vi "Speed of VIight FPGA_v2.vi"() -> ()   [LabVIEW 2026]
uses:
  <vilib>/eio/EIONode/EIONode.xnode
  <vilib>/rvi/eio/common/nirviEmuTemplateMethod_errors.vi
  <instrlib>/_niInstr/Basic Elements/v1/FPGA/niInstr Basic Elements v1 FPGA.lvlib
  <instrlib>/_niInstr/Basic Elements/v1/FPGA/Private/Count Up U16.vi
panel:
  out "Any Invalid press":bool
  out "Any Press":bool
  out "Any Valid press":bool
  out "Idle Loop":i32
  in  "Period":u16=100
  in  "Idle Pattern":u16[](array[numeric])=[0, 0, 0, 0, 0, 0, 0, 0, 0, 0, 0, 0, 0, 0, 0, 0, 0, 0, 0, 0, 0, 0, 0, 0, 0, 0, 0, 0, 0, 0, 0, 0, 0, 0, 0, 0, 0, 0, 0, 0, 0, 0, 0, 0, 0]
  out "Main Loop Complete":bool
  out "Player 2 Output 5":bool[](array[boolean])
  out "Player 1 Output 5":bool[](array[boolean])
  out "Initial 6 Random Numbers":u8[](array[numeric])
  out "Player 2 Bonus":u8
  out "Player 1 Bonus":u8
  in  "Max Bonus":u8=5
  in  "Bonus Threshold":u64=3000
  out "Intial Random Arrays":u8[](array[numeric])
  out "Player2 Input":bool[](array[boolean])
  out "Player1 Input":bool[](array[boolean])
  out "Player 2 Output 4":bool[](array[boolean])
  out "Player 2 Output 3":bool[](array[boolean])
  out "Player 2 Output 2":bool[](array[boolean])
  out "Player 2 Output 1":bool[](array[boolean])
  out "Player 1 Output 4":bool[](array[boolean])
  out "Player 1 Output 3":bool[](array[boolean])
  out "Player 1 Output 2":bool[](array[boolean])
  out "Player 2 Score":u32
  out "Player 2 Timer":u64
  out "Player 1 Score":u32
  out "Player 1 Timer":u64
  out "Main Loop":i32
  out "Closing Loop":i32
  out "Element to change 2":i32
  out "Element to change":i32
  out "Measured Main Loop Ticks":u32
  in  "Main Loop Timer":u32=1 caption="Main Loop Timer (uSec)"
  out "Player2 Output Number":u32
  out "Player1 Output Number":u32
  out "Initialized Array 2":bool[](array[boolean])
  out "Initialized Array 1":bool[](array[boolean])
  out "Random Number":u8
  in  "Random Number Max":u8=20
  out "Current State":i16
  out "Blue2":bool
  out "Green3":bool
  out "Green2":bool
  out "Blue1":bool
  out "Green1":bool
  out "Player 1 Output":bool[](array[boolean])
  in  "Game Length (s)":u32=45
  in  "Stop Closing Loop":bool
  in  "Stop Main Loop":bool
  in  "Stop Idle":bool
  in  "Global Stop":bool
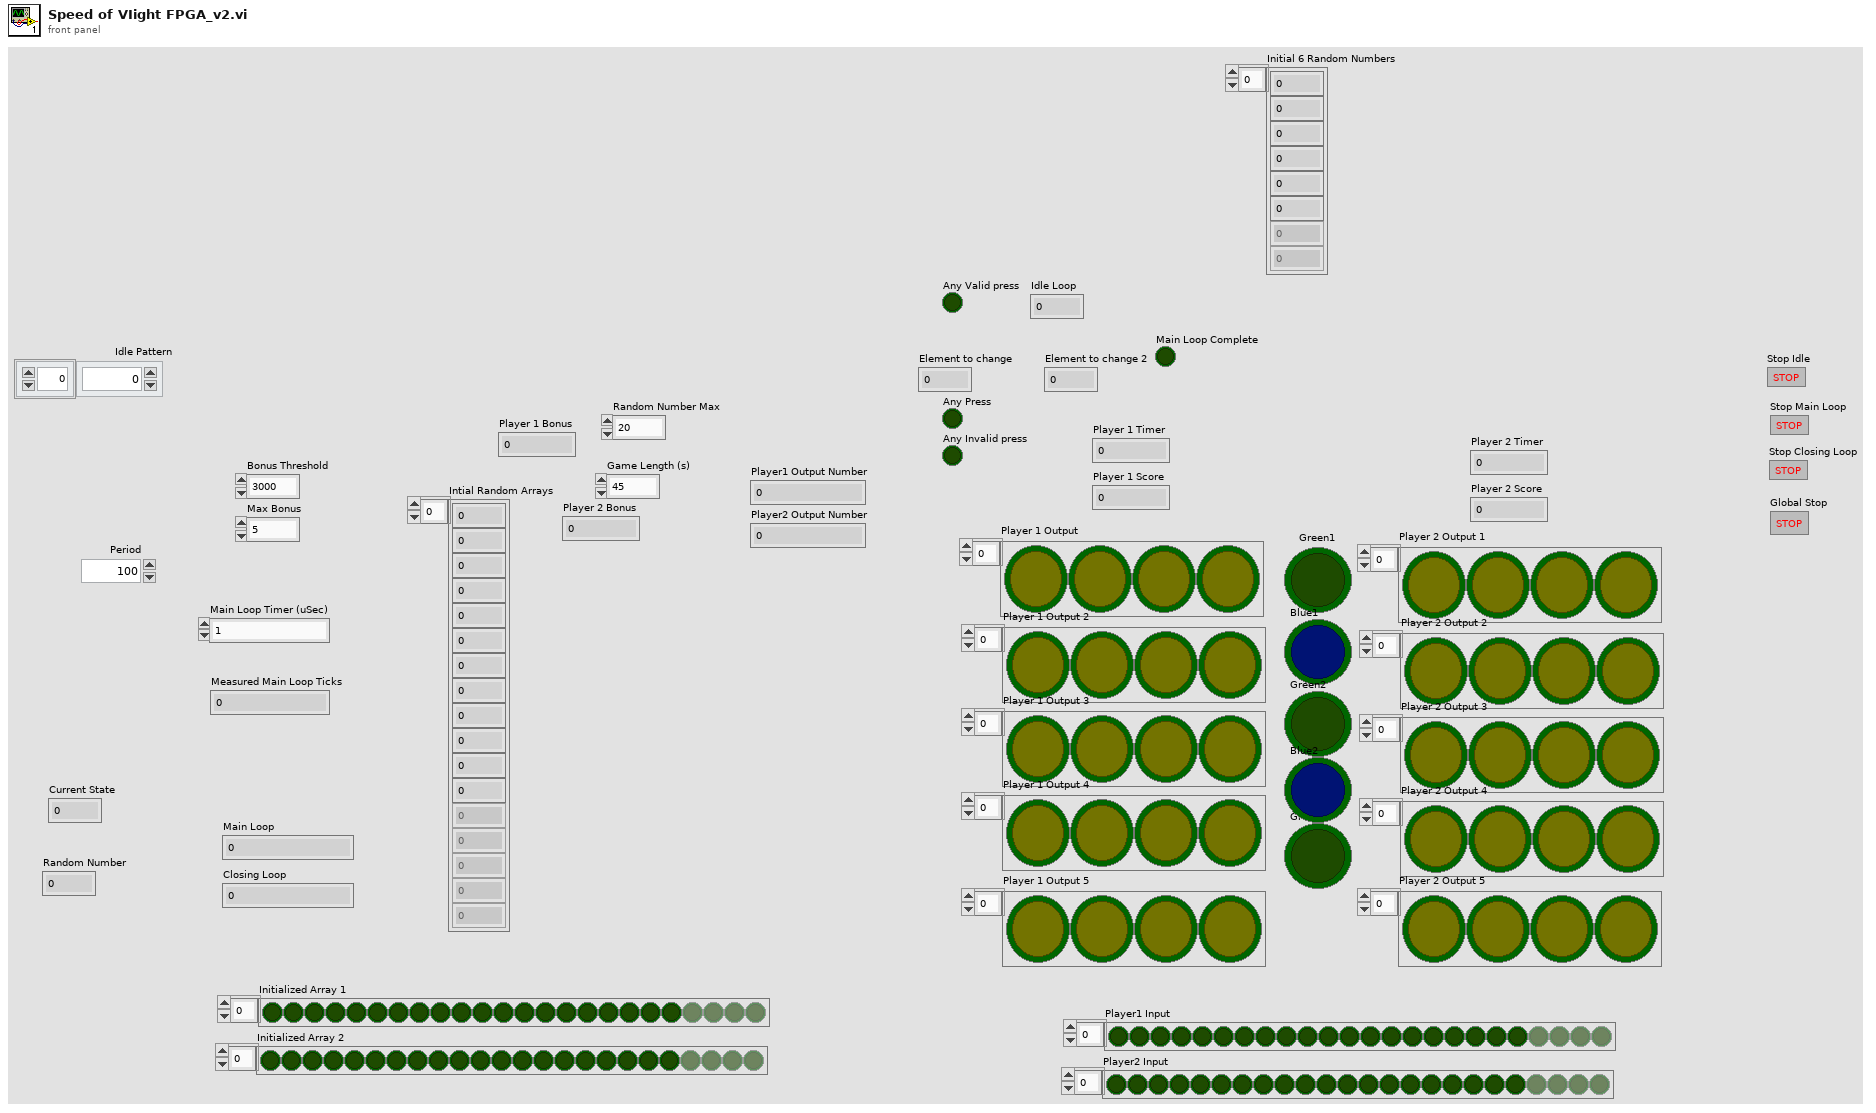
[diagram p1: front panel]
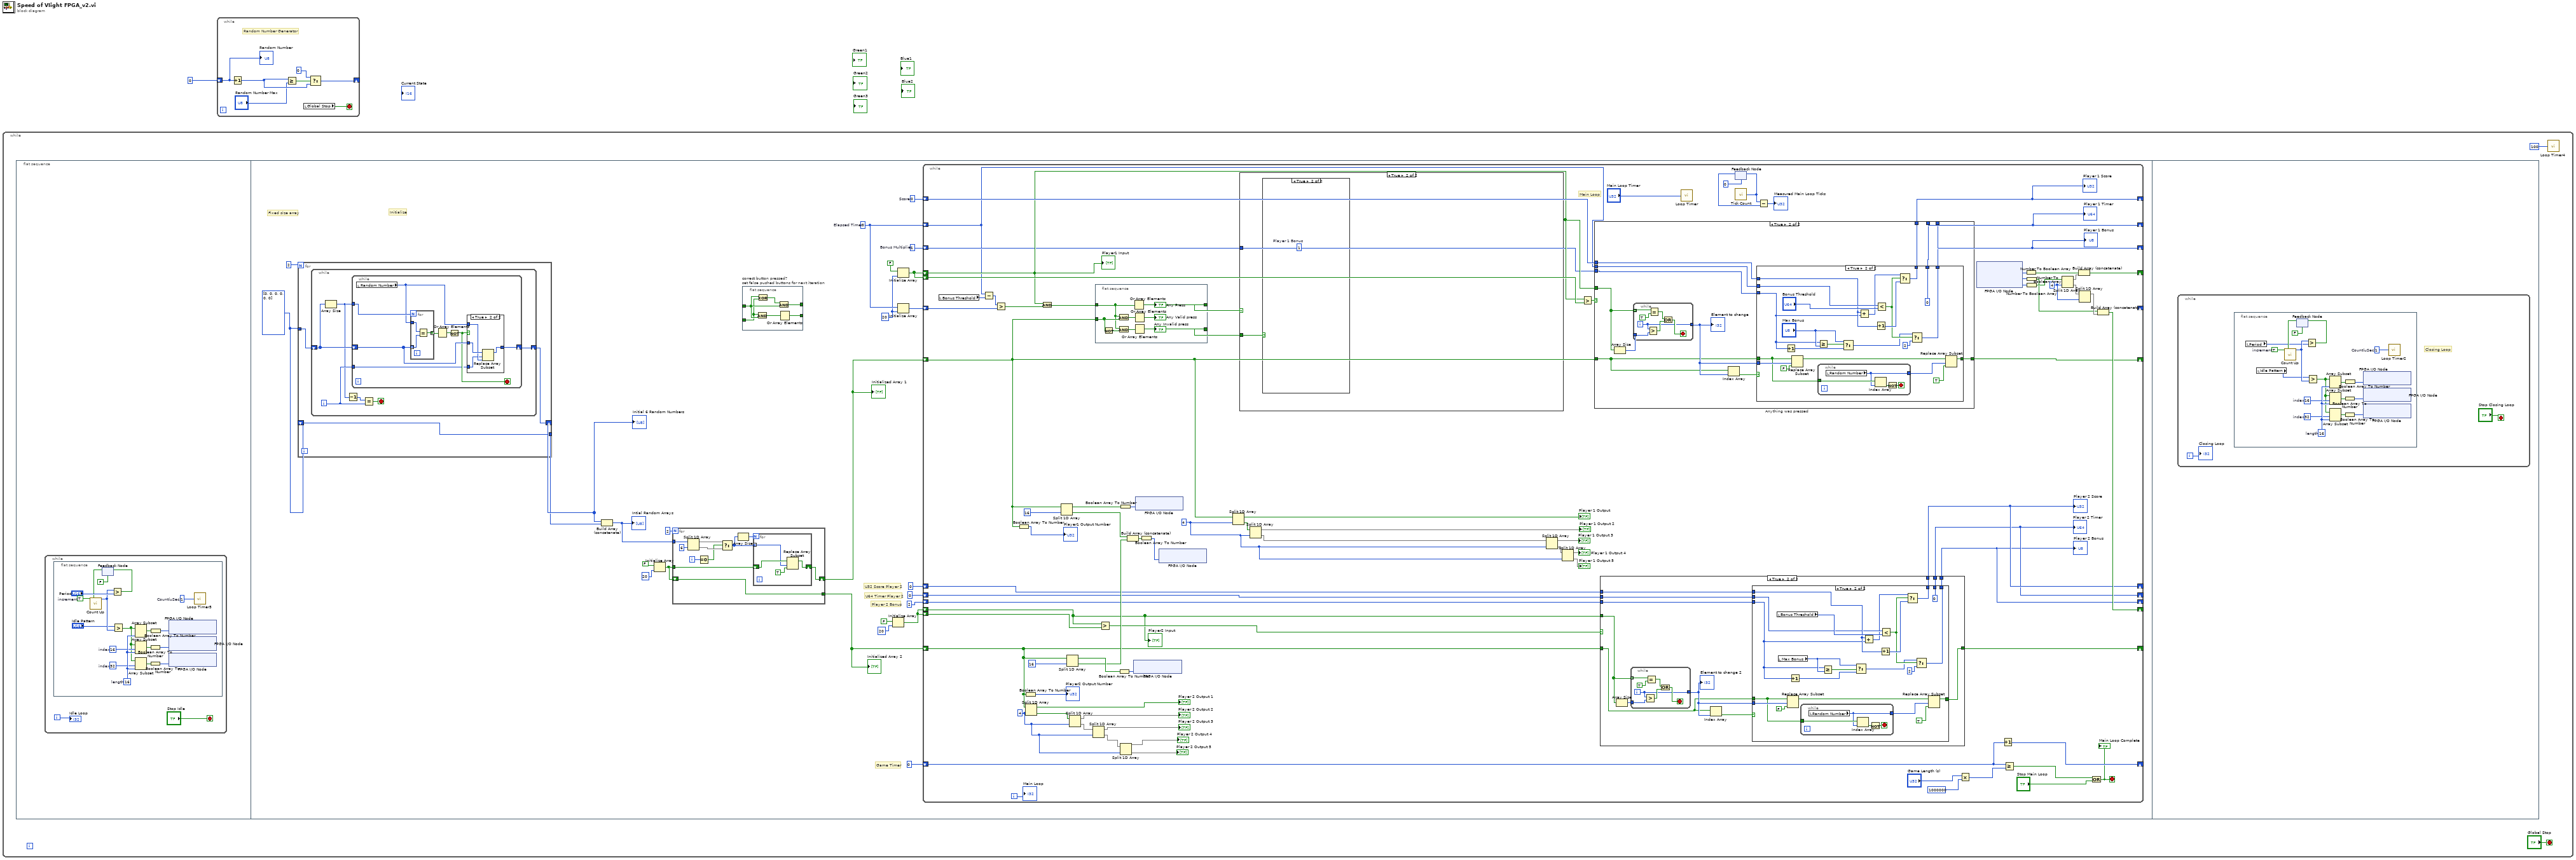
[diagram p0: block diagram]
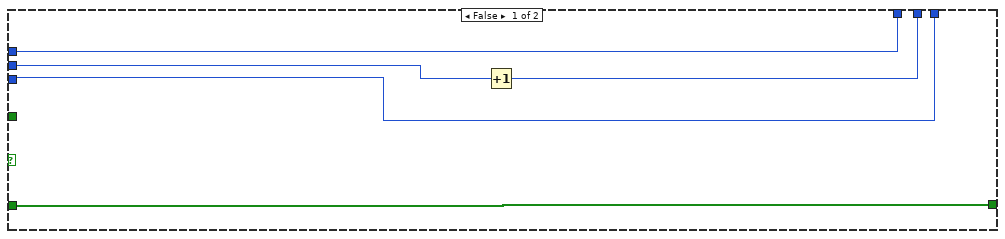
[diagram p5: hidden frame]
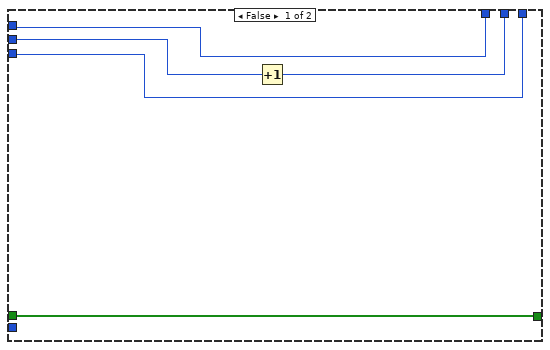
[diagram p6: hidden frame]
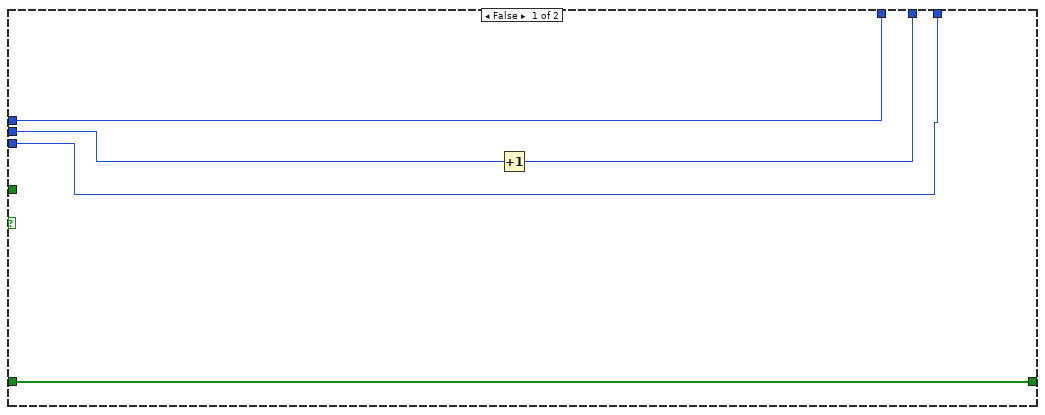
[diagram p7: hidden frame]
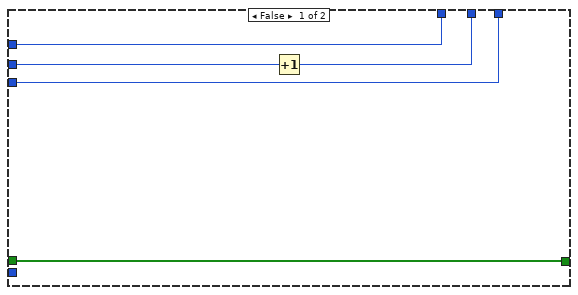
[diagram p8: hidden frame]
diagram:
  n1 = while {
    stop <- "Global Stop" stop-if-true
    n2 = flat-sequence {
      frame #0 {
        n3 = while {
          i -> [w4]
          stop <- "Stop Idle" stop-if-true
          n4 = flat-sequence {
            frame #0 {
              w10 = 32  # index
              w11 = 16  # index
              w12 = 16  # length
              w19 = u16 1  # Count(uSec)
              w22 = TRUE  # increment
              n5 = feedback #1(FALSE) -> (w18:bool)
              n6 = call-poly <instrlib>:"Count Up.vi"("increment"=w22, "reset"=w18) -> ("count out"=w17:u16)  [unwired: 13 in]
              n7 = Greater?(x=w17, y="Period") -> (0:w20:bool)
              n8 = feedback-in #1(w20) -> ()
              n9 = Greater?(x="Idle Pattern", y=w17) -> (0:w8:bool[])
              n10 = Array Subset(array=w8, length=w12) -> (w6:bool[])  [unwired: 1 in]
              n11 = Array Subset(array=w8, index=w11, length=w12) -> (w7:bool[])
              n12 = Array Subset(array=w8, index=w10, length=w12) -> (w9:bool[])
              n13 = Boolean Array To Number(Boolean array=w7) -> (number=w14:u16)
              n14 = Boolean Array To Number(Boolean array=w9) -> (number=w13:u16)
              n15 = Boolean Array To Number(Boolean array=w6) -> (number=w15:u16)
              n16 = xnode "FPGA I/O Node"("Bank-01/DO15:0"=w15) -> ()  [unwired: 1 in, 1 out]
              n17 = xnode "FPGA I/O Node"("Bank-02/DO15:0"=w14) -> ()  [unwired: 1 in, 1 out]
              n18 = xnode "FPGA I/O Node"("Bank-03/DO15:0"=w13) -> ()  [unwired: 1 in, 1 out]
              n19 = call "Loop Timer5"("Count(uSec)"=w19) -> ()  [unwired: 1 out]
            }
          }
          "Idle Loop" <- w4
        }
      }
      frame #1 {
        w25 = 20 ("dimension size")
        w40 = u8 1  # Bonus Multiplier
        w33 = u8[] [0, 0, 0, 0, 0, 0] ("Initial Random Numbers")
        w47 = u32 0  # Score
        w26 = u64 0  # Elapsed Timer
        # "Player 2 Bonus"
        # "Initialize"
        # "Fixed size array"
        # "Game Timer"
        # "U32 Score Player 2"
        # "U64 Timer Player 2"
        n20 = for {
          N: 2 -> [_]
          tunnel: w33 -> [w72]
          shift-right: [w71] -> w32
          shift-left: w33 -> [w70]
          tunnel: [w70] -> w31
          n21 = while {
            shift-right: [w75] -> w71
            shift-left: w72 -> [w76]
            i -> [w78]
            stop <- w77 stop-if-true
            n22 = Array Size(array=w76) -> (size(s)=w73:i32)
            n23 = Decrement(x=w73) -> (x-1=w74:i32)
            n24 = while {
              tunnel: w78 -> [w80]
              shift-right: [w81] -> w75
              shift-left: w76 -> [w83]
              tunnel: w73 -> [w86]
              stop <- w82 stop-if-true
              n25 = local read "Random Number"() -> (w79:u8)
              n26 = for {
                N: w86 -> [_]
                tunnel: w83 -> [w93] mode=indexing
                tunnel: w79 -> [w94]
                tunnel: [w92] -> w85 mode=indexing
                n27 = Equal?(x=w94, y=w93) -> (x = y?=w92:bool)
              }
              n28 = Or Array Elements(Boolean array=w85) -> (logical OR=w84:bool)
              n29 = Not(x=w84) -> (.not. x?=w82:bool)
              n30 = case shown="True" w82 {
                tunnel: w83 -> [w87 w91]
                tunnel: [w87 w90] -> w81
                tunnel: w79 -> [_ w89]
                tunnel: w80 -> [_ w88]
                frame False {
                }
                frame True {
                  n31 = Replace Array Subset(array=w91, new element=w89, index=w88) -> (w90:u8[])
                }
              }
            }
            n32 = Equal?(x=w74, y=w78) -> (x = y?=w77:bool)
          }
        }
        "Initial 6 Random Numbers" <- w32
        n33 = Build Array (concatenate)(w32, w31) -> (w30:u8[])
        "Intial Random Arrays" <- w30
        n34 = Initialize Array(FALSE ("Boolean"), 20 ("dimension size")) -> (w34:bool[])
        n35 = for {
          N: 2 -> [_]
          tunnel: w34 -> [w64]
          tunnel: w30 -> [w62]
          shift-right: [w65] -> w29
          shift-left: w34 -> [w55]
          tunnel: [w55] -> w28
          i -> [w58]
          n36 = Split 1D Array(array=w62, index=6) -> (first subarray=w59:u8[], second subarray=w60:u8[])
          n37 = Equal To 0?(x=w58) -> (x = 0?=w57:bool)
          n38 = Select(t=w59, s=w57, f=w60) -> (s? t:f=w56:u8[])
          n39 = Array Size(array=w56) -> (size(s)=w63:i32)
          n40 = for {
            N: w63 -> [_]
            tunnel: w56 -> [w66] mode=indexing
            shift-right: [w69] -> w65
            shift-left: w64 -> [w68]
            n41 = Replace Array Subset(array=w68, new element=TRUE ("new element/subarray"), index=w66) -> (w69:bool[])
          }
        }
        "Initialized Array 1" <- w29
        "Initialized Array 2" <- w28
        n42 = flat-sequence "correct button pressed?\nset false pushed buttons for next iteration" {
          tunnel: [w53] -> _
          tunnel: _ -> [w51]
          tunnel: _ -> [w50]
          tunnel: [w49] -> _
          frame #0 {
            n43 = And(x=w50, y=w51) -> (x .and. y?=w52:bool)
            n44 = Exclusive Or(1:w50, 2:w51) -> (0:w54:bool)
            n45 = And(x=w54, y=w51) -> (x .and. y?=w53:bool)
            n46 = Or Array Elements(Boolean array=w52) -> (logical OR=w49:bool)
          }
        }
        n47 = Initialize Array(FALSE ("Boolean"), 20 ("dimension size")) -> (w35:bool[])
        n48 = Initialize Array(FALSE ("Boolean"), w25) -> (w38:bool[])
        n49 = Initialize Array(w26, w25) -> (w24:u64[])
        n50 = while {
          shift-right: [w124] -> _
          shift-left: w26 -> [w99]
          shift-right: [w118] -> _
          shift-left: u64 0 -> [w122]
          shift-right: [w125] -> _
          shift-left: w47 -> [w126]
          shift-right: [w119] -> _
          shift-left: u32 0 -> [w120]
          shift-right: [w177] -> _
          shift-left: u32 0 -> [w178]
          shift-right: [w147] -> _
          shift-left: w29 -> [w105]
          shift-right: [w144] -> _
          shift-left: w28 -> [w138]
          shift-right: [w152] -> _
          shift-left: w38 -> [w104]
          shift-right: [w151] -> _
          shift-left: w35 -> [w127]
          shift-left: w38 -> [w150]
          shift-left: w35 -> [w146]
          shift-right: [w123] -> _
          shift-left: w40 -> [w101]
          shift-right: [w117] -> _
          shift-left: u8 2 -> [w121]
          shift-right: _ -> [_]
          shift-left: w24 -> [w98]
          i -> [w140]
          stop <- w106 stop-if-true
          w107 = 4 ("index")
          w114 = 4 ("index")
          w158 = 4 ("index")
          # "Main Loop"
          n51 = local read "Bonus Threshold"() -> (w96:u64)
          n52 = Subtract(x=w99, y=w96) -> (x-y=w97:u64)
          n53 = Greater?(x=w97, y=w98) -> (0:w95:bool[])
          n54 = Boolean Array To Number(Boolean array=w105) -> (number=→"Player1 Output Number":u32)
          n55 = Boolean Array To Number(Boolean array=w138) -> (number=→"Player2 Output Number":u32)
          n56 = Split 1D Array(array=w138, index=w114) -> (first subarray=→"Player 2 Output 1":bool[], second subarray=w136:bool[])
          n57 = And(x=w104, y=w95) -> (x .and. y?=w100:bool[])
          n58 = Split 1D Array(array=w105, index=16) -> (first subarray=w148:bool[], second subarray=w168:bool[])
          n59 = Split 1D Array(array=w138, index=16) -> (first subarray=w171:bool[], second subarray=w167:bool[])
          n60 = Split 1D Array(array=w136, index=w114) -> (first subarray=→"Player 2 Output 2":bool[], second subarray=w134:bool[])
          n61 = Split 1D Array(array=w134, index=w114) -> (first subarray=→"Player 2 Output 3":bool[], second subarray=w112:bool[])
          n62 = flat-sequence {
            tunnel: w105 -> [w186]
            tunnel: w100 -> [w185]
            tunnel: [w182] -> w103
            tunnel: [w181] -> w102
            frame #0 {
              n63 = Not(x=w186) -> (.not. x?=w184:bool[])
              n64 = And(x=w185, y=w186) -> (x .and. y?=w188:bool[])
              n65 = And(x=w185, y=w184) -> (x .and. y?=w183:bool[])
              n66 = Or Array Elements(Boolean array=w185) -> (logical OR=w182:bool)
              "Any Press" <- w182
              n67 = Or Array Elements(Boolean array=w188) -> (logical OR=→"Any Valid press":bool)
              n68 = Or Array Elements(Boolean array=w183) -> (logical OR=w181:bool)
              "Any Invalid press" <- w181
            }
          }
          n69 = Greater?(x=w127, y=w146) -> (0:w145:bool)
          n70 = Boolean Array To Number(Boolean array=w171) -> (number=w170:u32)
          n71 = Boolean Array To Number(Boolean array=w148) -> (number=w173:u32)
          n72 = Split 1D Array(array=w112, index=w114) -> (first subarray=→"Player 2 Output 4":bool[], second subarray=→"Player 2 Output 5":bool[])
          n73 = Build Array (concatenate)(w168, w167) -> (w166:bool[])
          n74 = xnode "FPGA I/O Node"("Bank-02/DO15:0"=w170) -> ()  [unwired: 1 in, 1 out]
          n75 = xnode "FPGA I/O Node"("Bank-01/DO15:0"=w173) -> ()  [unwired: 1 in, 1 out]
          n76 = Boolean Array To Number(Boolean array=w166) -> (number=w165:u32)
          n77 = xnode "FPGA I/O Node"("Bank-03/DO15:0"=w165) -> ()  [unwired: 1 in, 1 out]
          n78 = Split 1D Array(array=w105, index=w107) -> (first subarray=→"Player 1 Output":bool[], second subarray=w132:bool[])
          n79 = case shown="True" w103 {
            tunnel: w102 -> [_ w180]
            tunnel: w101 -> [_ _]
            frame False {
            }
            frame True {
              n80 = case shown="True" w180 {
                frame False {
                }
                frame True {
                  (unwired) u8 1  # Player 1 Bonus
                }
              }
            }
          }
          n81 = Split 1D Array(array=w132, index=w107) -> (first subarray=→"Player 1 Output 2":bool[], second subarray=w131:bool[])
          n82 = Split 1D Array(array=w131, index=w107) -> (first subarray=→"Player 1 Output 3":bool[], second subarray=w110:bool[])
          n83 = Split 1D Array(array=w110, index=w107) -> (first subarray=→"Player 1 Output 4":bool[], second subarray=→"Player 1 Output 5":bool[])
          n84 = Greater?(x=w104, y=w150) -> (0:w149:bool)
          n85 = case "Anything was pressed" shown="True" w149 {
            tunnel: [w248 w260] -> w147
            tunnel: w104 -> [_ w257]
            tunnel: w105 -> [w248 w255]
            tunnel: w99 -> [w246 w251]
            tunnel: [w245 w253] -> w124
            tunnel: w126 -> [w247 w252]
            tunnel: [w247 w254] -> w125
            tunnel: w101 -> [w244 w250]
            tunnel: [w244 w249] -> w123
            frame False {
              n86 = Increment(x=w246) -> (x+1=w245:u64)
            }
            frame True {
              n87 = Array Size(array=w257) -> (size(s)=w256:i32)
              n88 = while {
                tunnel: w257 -> [w298] mode=indexing
                tunnel: w256 -> [w294]
                tunnel: [w292] -> w259
                i -> [w292]
                stop <- w295 stop-if-true
                n89 = Greater?(x=w292, y=w294) -> (0:w293:bool)
                n90 = Equal?(x=w298, y=TRUE ("element")) -> (x = y?=w296:bool)
                n91 = Or(x=w296, y=w293) -> (x .or. y?=w295:bool)
              }
              "Element to change" <- w259
              n92 = Index Array(array=w255, index=w259) -> (element=w258:bool)
              n93 = case shown="True" w258 {
                tunnel: w259 -> [_ w287]
                tunnel: [w265 w283] -> w260
                tunnel: w255 -> [w265 w281]
                tunnel: w252 -> [w264 w268]
                tunnel: w251 -> [w263 w279]
                tunnel: [w264 w277] -> w254
                tunnel: [w262 u64 0] -> w253
                tunnel: w250 -> [w261 w267]
                tunnel: [w261 w274] -> w249
                frame False {
                  n94 = Increment(x=w263) -> (x+1=w262:u64)
                }
                frame True {
                  n95 = Increment(x=w267) -> (x+1=w270:u8)
                  n96 = Replace Array Subset(array=w281, new element=FALSE ("new element/subarray"), index=w287) -> (w285:bool[])
                  n97 = Greater Or Equal?(x=w267, y="Max Bonus") -> (x >= y?=w272:bool)
                  n98 = while {
                    tunnel: [w288] -> w282
                    tunnel: w281 -> [w291]
                    stop <- w289 stop-if-true
                    n99 = local read "Random Number"() -> (w288:u8)
                    n100 = Index Array(array=w291, index=w288) -> (element=w290:bool)
                    n101 = Not(x=w290) -> (.not. x?=w289:bool)
                  }
                  n102 = Select(t="Max Bonus", s=w272, f=w270) -> (s? t:f=w269:u8)
                  n103 = Add(x=w268, y=w267) -> (x+y=w266:u32)
                  n104 = Increment(x=w268) -> (x+1=w278:u32)
                  n105 = Less?(x=w279, y="Bonus Threshold") -> (x < y?=w276:bool)
                  n106 = Select(t=w266, s=w276, f=w278) -> (s? t:f=w277:u32)
                  n107 = Select(t=w269, s=w276, f=u8 2) -> (s? t:f=w274:u8)
                  n108 = Replace Array Subset(array=w285, new element=TRUE ("new element/subarray"), index=w282) -> (w283:bool[])
                }
              }
            }
          }
          "Player 1 Timer" <- w124
          "Player 1 Score" <- w125
          "Player 1 Bonus" <- w123
          n109 = case shown="True" w145 {
            tunnel: [w193 w201] -> w144
            tunnel: w127 -> [_ w203]
            tunnel: w138 -> [w193 w200]
            tunnel: w122 -> [w191 w198]
            tunnel: w121 -> [w189 w197]
            tunnel: w120 -> [w192 w199]
            tunnel: [w192 w195] -> w119
            tunnel: [w190 w196] -> w118
            tunnel: [w189 w194] -> w117
            frame False {
              n110 = Increment(x=w191) -> (x+1=w190:u64)
            }
            frame True {
              n111 = Array Size(array=w203) -> (size(s)=w202:i32)
              n112 = while {
                tunnel: w203 -> [w243] mode=indexing
                tunnel: w202 -> [w239]
                tunnel: [w237] -> w205
                i -> [w237]
                stop <- w240 stop-if-true
                n113 = Greater?(x=w237, y=w239) -> (0:w238:bool)
                n114 = Equal?(x=w243, y=TRUE ("element")) -> (x = y?=w241:bool)
                n115 = Or(x=w241, y=w238) -> (x .or. y?=w240:bool)
              }
              "Element to change 2" <- w205
              n116 = Index Array(array=w200, index=w205) -> (element=w204:bool)
              n117 = case shown="True" w204 {
                tunnel: w205 -> [_ w232]
                tunnel: [w210 w228] -> w201
                tunnel: w200 -> [w210 w226]
                tunnel: w199 -> [w206 w218]
                tunnel: w198 -> [w209 w213]
                tunnel: w197 -> [w207 w211]
                tunnel: [w208 u64 0] -> w196
                tunnel: [w207 w216] -> w194
                tunnel: [w206 w215] -> w195
                frame False {
                  n118 = Increment(x=w209) -> (x+1=w208:u64)
                }
                frame True {
                  n119 = local read "Bonus Threshold"() -> (w220:u64)
                  n120 = local read "Max Bonus"() -> (w219:u8)
                  n121 = Replace Array Subset(array=w226, new element=FALSE ("new element/subarray"), index=w232) -> (w230:bool[])
                  n122 = Increment(x=w211) -> (x+1=w214:u8)
                  n123 = while {
                    tunnel: [w233] -> w227
                    tunnel: w226 -> [w236]
                    stop <- w234 stop-if-true
                    n124 = local read "Random Number"() -> (w233:u8)
                    n125 = Index Array(array=w236, index=w233) -> (element=w235:bool)
                    n126 = Not(x=w235) -> (.not. x?=w234:bool)
                  }
                  n127 = Greater Or Equal?(x=w211, y=w219) -> (x >= y?=w222:bool)
                  n128 = Select(t=w219, s=w222, f=w214) -> (s? t:f=w221:u8)
                  n129 = Add(x=w218, y=w211) -> (x+y=w212:u32)
                  n130 = Increment(x=w218) -> (x+1=w225:u32)
                  n131 = Less?(x=w213, y=w220) -> (x < y?=w224:bool)
                  n132 = Select(t=w212, s=w224, f=w225) -> (s? t:f=w215:u32)
                  n133 = Select(t=w221, s=w224, f=u8 2) -> (s? t:f=w216:u8)
                  n134 = Replace Array Subset(array=w230, new element=TRUE ("new element/subarray"), index=w227) -> (w228:bool[])
                }
              }
            }
          }
          "Player 2 Timer" <- w118
          "Player 2 Score" <- w119
          "Player 2 Bonus" <- w117
          n135 = call "Loop Timer"("Count(uSec)"="Main Loop Timer") -> ()  [unwired: 1 out]
          n136 = feedback #2(u32 0) -> (w155:u32)
          n137 = call "Tick Count"() -> ("Tick Count(Ticks)"=w154:u32)
          n138 = feedback-in #2(w154) -> ()
          n139 = Subtract(x=w154, y=w155) -> (x-y=→"Measured Main Loop Ticks":u32)
          n140 = Multiply(x="Game Length (s)", y=u32 1000000) -> (x*y=w141:u32)
          n141 = xnode "FPGA I/O Node"() -> ("Bank-01/DI15:0"=w164:u16, "Bank-02/DI15:0"=w163:u16, "Bank-03/DI15:0"=w162:u16)  [unwired: 3 in, 3 out]
          n142 = Increment(x=w178) -> (x+1=w177:u32)
          n143 = Greater Or Equal?(x=w178, y=w141) -> (x >= y?=w176:bool)
          n144 = Number To Boolean Array(number=w164) -> (Boolean array=w160:bool[])
          n145 = Number To Boolean Array(number=w163) -> (Boolean array=w115:bool[])
          n146 = Number To Boolean Array(number=w162) -> (Boolean array=w116:bool[])
          n147 = Split 1D Array(array=w116, index=w158) -> (first subarray=w159:bool[], second subarray=w157:bool[])
          n148 = Build Array (concatenate)(w160, w159) -> (w152:bool[])
          n149 = Split 1D Array(array=w157, index=w158) -> (first subarray=w156:bool[])  [unwired: 1 out]
          n150 = Or(x=w176, y="Stop Main Loop") -> (x .or. y?=w106:bool)
          "Main Loop Complete" <- w106
          n151 = Build Array (concatenate)(w115, w156) -> (w151:bool[])
          "Main Loop" <- w140
          "Player1 Input" <- w104
          "Player2 Input" <- w127
        }
      }
      frame #2 {
        n152 = while {
          i -> [w299]
          stop <- "Stop Closing Loop" stop-if-true
          # "Closing Loop"
          n153 = flat-sequence {
            frame #0 {
              w307 = 32  # index
              w308 = 16  # index
              w309 = 16  # length
              w315 = u16 1  # Count(uSec)
              w318 = TRUE  # increment
              n154 = local read "Period"() -> (w301:u16)
              n155 = local read "Idle Pattern"() -> (w302:u16[])
              n156 = feedback #3(FALSE) -> (w314:bool)
              n157 = call-poly <instrlib>:"Count Up.vi"("increment"=w318, "reset"=w314) -> ("count out"=w313:u16)  [unwired: 13 in]
              n158 = Greater?(x=w313, y=w301) -> (0:w316:bool)
              n159 = feedback-in #3(w316) -> ()
              n160 = Greater?(x=w302, y=w313) -> (0:w305:bool[])
              n161 = Array Subset(array=w305, length=w309) -> (w303:bool[])  [unwired: 1 in]
              n162 = Array Subset(array=w305, index=w308, length=w309) -> (w304:bool[])
              n163 = Array Subset(array=w305, index=w307, length=w309) -> (w306:bool[])
              n164 = Boolean Array To Number(Boolean array=w304) -> (number=w311:u16)
              n165 = Boolean Array To Number(Boolean array=w306) -> (number=w310:u16)
              n166 = Boolean Array To Number(Boolean array=w303) -> (number=w312:u16)
              n167 = xnode "FPGA I/O Node"("Bank-01/DO15:0"=w312) -> ()  [unwired: 1 in, 1 out]
              n168 = xnode "FPGA I/O Node"("Bank-02/DO15:0"=w311) -> ()  [unwired: 1 in, 1 out]
              n169 = xnode "FPGA I/O Node"("Bank-03/DO15:0"=w310) -> ()  [unwired: 1 in, 1 out]
              n170 = call "Loop Timer2"("Count(uSec)"=w315) -> ()  [unwired: 1 out]
            }
          }
          "Closing Loop" <- w299
        }
      }
    }
    n171 = call "Loop Timer4"("Count(mSec)"=u32 100 ("millisecond multiple")) -> ()  [unwired: 1 out]
  }
  n172 = while {
    shift-right: [w323] -> _
    shift-left: u8 0 -> [w325]
    stop <- w319 stop-if-true
    # "Random Number Generator"
    n173 = Increment(x=w325) -> (x+1=w322:u8)
    n174 = Greater Or Equal?(x=w322, y="Random Number Max") -> (x >= y?=w321:bool)
    n175 = local read "Global Stop"() -> (w319:bool)
    n176 = Select(t=u8 0, s=w321, f=w322) -> (s? t:f=w323:u8)
    "Random Number" <- w325
  }
